vi "Get Plugin Configuration.vi"(8 "error in (no error)":errorcluster, 11 "Component Configuration in":refnum<class "Component Configurations.lvclass">) -> (0 "error out":errorcluster, 2 "Plugin Configuration":refnum<class "Configuration.lvclass">, 3 "Component Configuration out":refnum<class "Component Configurations.lvclass">)   [LabVIEW 2021, in "DSF Core.lvlib" / "Component Configurations.lvclass"]
uses:
  Component Configurations.lvclass
  Configuration/Configuration.lvclass
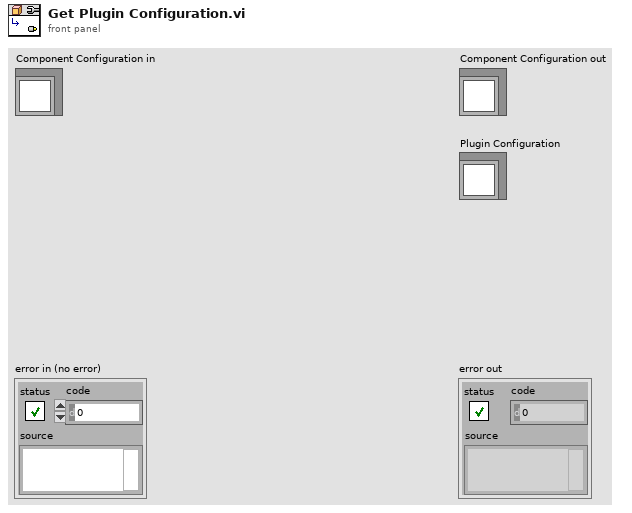
[diagram p1: front panel]
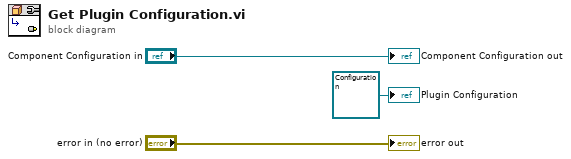
[diagram p0: block diagram]
diagram:
  "error out" <- "error in (no error)"
  "Component Configuration out" <- "Component Configuration in"
  "Plugin Configuration" <- refnum<class "Configuration.lvclass"> refnum ("Plugin Configuration")
